vi "test Get Base 8.vi"(11 "Test Case In":refnum<class "test EDS.lvclass">) -> (0 "error out":errorcluster, 3 "Test Case Out":refnum<class "test EDS.lvclass">)   [LabVIEW 2024, in "test EDS.lvclass"]
uses:
  test EDS.lvclass
  <vilib>/Astemes/LUnit/Test Case.lvclass/Test Case.ctl
  <vilib>/Astemes/LUnit/Append Fail Result.vi
  <vilib>/Astemes/LUnit/Append Pass Result.vi
  <vilib>/Astemes/LUnit/Run In UI.vi
  <vilib>/Utility/error.llb/Clear Errors.vi
  test EDS.lvclass/test EDS.ctl
  Core/EDS.lvlib
  <vilib>/Astemes/LUnit/Test Case.lvclass
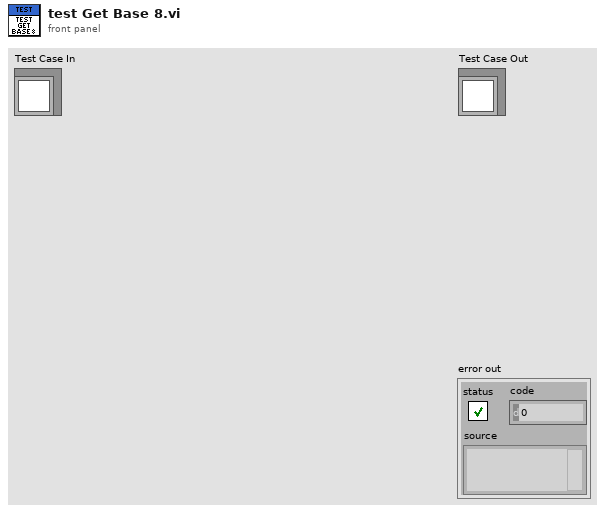
[diagram p1: front panel]
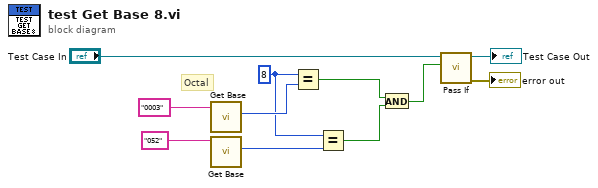
[diagram p0: block diagram]
diagram:
  w4 = u8 8
  # "Octal"
  n1 = call "Get Base.vi"("Default Value"="0003") -> ("Number Base"=w6:u8)  [unwired: 9 in, 1 out]
  n2 = call "Get Base.vi"("Default Value"="052") -> ("Number Base"=w5:u8)  [unwired: 9 in, 1 out]
  n3 = Equal?(x=w4, y=w6) -> (x = y?=w3:bool)
  n4 = Equal?(x=w4, y=w5) -> (x = y?=w2:bool)
  n5 = And(x=w3, y=w2) -> (x .and. y?=w1:bool)
  n6 = call <vilib>:"Pass If.vi"("Pass?"=w1, "LUnit Test Case In"="Test Case In") -> ("error out"=→"error out":errorcluster, "LUnit Test Case Out"=→"Test Case Out":refnum<class "test EDS.lvclass">)  [unwired: 8 in]
